vi "Is Allowed File Type.vi"(8 "error in (no error)":errorcluster, 10 "y":string[](array[string]), 11 "Path":path) -> (0 "error out":errorcluster)   [LabVIEW 2020, in "G-AI Core.lvlib"]
uses:
  G-AI Core.lvlib
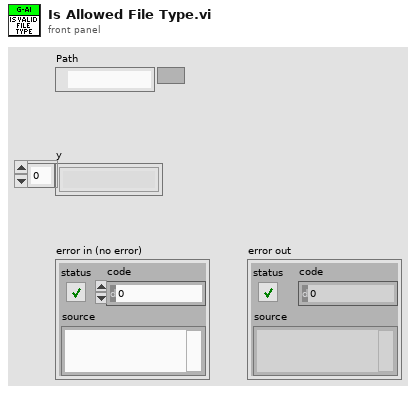
[diagram p1: front panel]
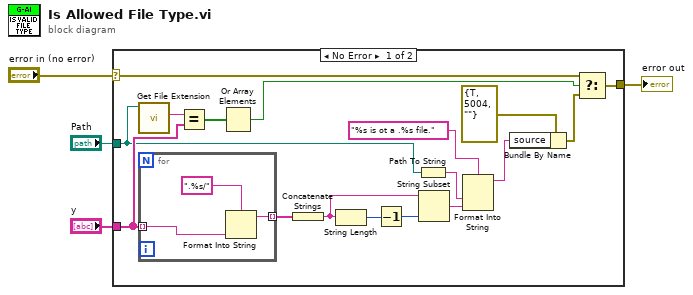
[diagram p0: block diagram]
diagram:
  n1 = case shown="No Error" "error in (no error)" {
    selector: "error in (no error)" -> [w5 w25]
    tunnel: [w21 w25] -> w4
    tunnel: "y" -> [w15 _]
    tunnel: "Path" -> [w12 _]
    frame No Error {
      n2 = call <vilib>:"Get File Extension.vi"("file"=w12) -> ("lowercase file extension"=w6:string)  [unwired: 6 in, 4 out]
      n3 = for {
        tunnel: w15 -> [w24] mode=indexing
        tunnel: [w22] -> w16 mode=indexing
        n4 = Format Into String(format string=".%s/", w24) -> (resulting string=w22:string)  [unwired: 2 in, 1 out]
      }
      n5 = Equal?(x=w6, y=w15) -> (x = y?=w7:bool[])
      n6 = Or Array Elements(Boolean array=w7) -> (logical OR=w14:bool)
      n7 = Concatenate Strings(w16) -> (w17:string)
      n8 = String Length(string=w17) -> (length=w18:i32)
      n9 = Decrement(x=w18) -> (x-1=w19:i32)
      n10 = Path To String(path=w12) -> (string=w13:string)
      n11 = String Subset(string=w17, length (rest)=w19) -> (substring=w20:string)  [unwired: 1 in]
      n12 = Format Into String(format string="%s is ot a .%s file.", w13, w20) -> (resulting string=w10:string)  [unwired: 2 in, 1 out]
      n13 = Bundle By Name(cluster=errorcluster {"status"=TRUE, "code"=5004, "source"=""} ("f"), "source"=w10) -> (w9:errorcluster)
      n14 = Select(t=w5, s=w14, f=w9) -> (s? t:f=w21:errorcluster)
    }
    frame Error {
    }
  }
  "error out" <- w4
